vi "Workspace.Channels.Create.vi"(11 "CD Path":string) -> (2 "Read Channels":string[](array[string]), 3 "Command Channel":string)   [LabVIEW 2019, in "Diagnostics Workspace Shared.lvlib"]
uses:
  Diagnostics Workspace Shared.lvlib
  Addon/Addon Shared/SubVIs/Constants.vi
  Addon/Addon Shared/Diagnostics Addon Shared.lvlib
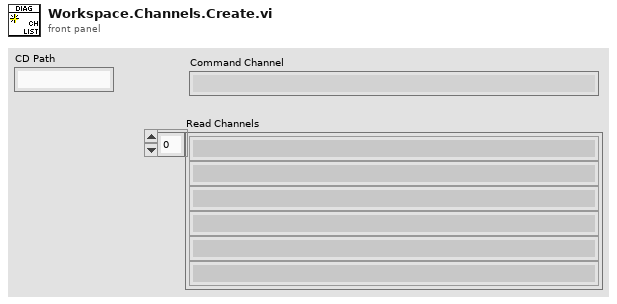
[diagram p1: front panel]
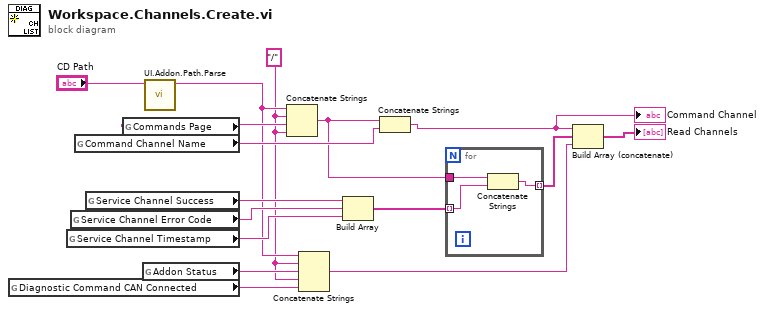
[diagram p0: block diagram]
diagram:
  w3 = "/" ("string")
  n1 = global read "Constants.vi" "Diagnostic Command CAN Connected"() -> (w5:string)
  n2 = global read "Constants.vi" "Service Channel Timestamp"() -> (w7:string)
  n3 = global read "Constants.vi" "Service Channel Error Code"() -> (w14:string)
  n4 = global read "Constants.vi" "Command Channel Name"() -> (w11:string)
  n5 = global read "Constants.vi" "Service Channel Success"() -> (w13:string)
  n6 = global read "Constants.vi" "Commands Page"() -> (w8:string)
  n7 = global read "Constants.vi" "Addon Status"() -> (w6:string)
  n8 = call "UI.Addon.Path.Parse.vi"("Cached Addon Path"="CD Path") -> ("Addon Path"=w4:string)  [unwired: 6 in, 4 out]
  n9 = Concatenate Strings(w4, w3, w8, w3) -> (w1:string)
  n10 = Concatenate Strings(w4, w3, w6, w3, w5) -> (w2:string)
  n11 = Build Array(w13, w14, w7) -> (w15:string[])
  n12 = Concatenate Strings(w1, w11) -> (w16:string)
  "Command Channel" <- w16
  n13 = for {
    tunnel: w1 -> [w19]
    tunnel: w15 -> [w17] mode=indexing
    tunnel: [w18] -> w12 mode=indexing
    n14 = Concatenate Strings(w19, w17) -> (w18:string)
  }
  n15 = Build Array (concatenate)(w16, w12, w2) -> (→"Read Channels":string[])
